vi "Event Handler.vi"(0 "uService Template in":refnum<class "TCP Writer.lvclass">, 5 "Event type":T1=enum."Message", 7 "Item Name":string, 9 "Data":variant, 11 "error in (no error)":errorcluster) -> (4 "uService Template out":refnum<class "TCP Writer.lvclass">, 15 "error out":errorcluster)   [LabVIEW 2026, in "TALOS.lvlib" / "TCP Writer.lvlib" / "TCP Writer.lvclass"]
uses:
  TCP Writer.lvclass
  C:/LabVIEW Code/TALOS/talos/Father of all uServices/Father of all uServices/Father of all uServices.lvclass
  Father of all uServices/Father of all uServices/Event Handler Items.ctl
  Ancestor/Ancestor/Ancestor.lvclass/Ancestor.ctl
  TCP Writer Consumer Case Selector.ctl
  Father of all uServices/Father of all uServices Messages/Consumer Msg/Consumer Msg.lvclass/Consumer Msg.ctl
  FGV/Error Memory/Get Error Description.vi
  Support VIs/Get PC name.vi
  Ancestor/Ancestor/Read ID.vi
  Support VIs/Get Class Name.vi
  <vilib>/Utility/error.llb/Clear Errors.vi
  Father of all uServices/Father of all uServices Messages/Consumer Msg/Send Consumer.vi
  Support VIs/Substitute Error.vi
  FGV/Error Memory/Error Memory Core.vi
  <vilib>/AdvancedString/Delimited String to 1D String Array.vi
  <vilib>/AdvancedString/Delimited String to 1D String Array (string).vi
  Support VIs/Circus Root Path.vi
  FGV/Error Memory/Error Crt Lvl checker.vi
  FGV/Error Memory/Error Memory Core.vi/40c8088d-b597-4017-91af-faa98e00292e.vi
  FGV/Error Memory/Error Memory Core.vi/d4a3ab98-063c-4e44-b43d-fbdcfe6c2be2.vi
  Father of all uServices/Father of all uServices/Father of all uServices.lvclass
  C:/LabVIEW Code/TALOS/builds/Actor Framework PPL/Actor Framework.lvlibp/1abvi3w/vi.lib/ActorFramework/Actor/Actor.lvclass
  Support VIs/Global Memory.vi
  <vilib>/Utility/LVClass/Get LV Class Name.vi
  Support VIs/Is in Packed Library.vi
  Support VIs/TALOS Root path.vi
  Support VIs/Read CSV worksheet.vi
  Support VIs/Global Constants.vi
  <vilib>/Utility/error.llb/General Error Handler.vi
  builds/Actor Framework PPL/Actor Framework.lvlibp/1abvi3w/vi.lib/ActorFramework/Actor/Read Self Enqueuer.vi
  <userlib>/_OpenG.lib/lvdata/lvdata.llb/Get Strings from Enum__ogtk.vi
  builds/Actor Framework PPL/Actor Framework.lvlibp/1abvi3w/vi.lib/ActorFramework/Message Enqueuer/Enqueue.vi
  Support VIs/Error Log.vi
  Ancestor/Ancestor/Ancestor.lvclass
  <vilib>/Comparison/Equal/Equal Functor/Equal Functor.lvclass
  Father of all uServices/Father of all uServices Messages/Consumer Msg/Consumer Msg.lvclass
  TALOS.lvlib
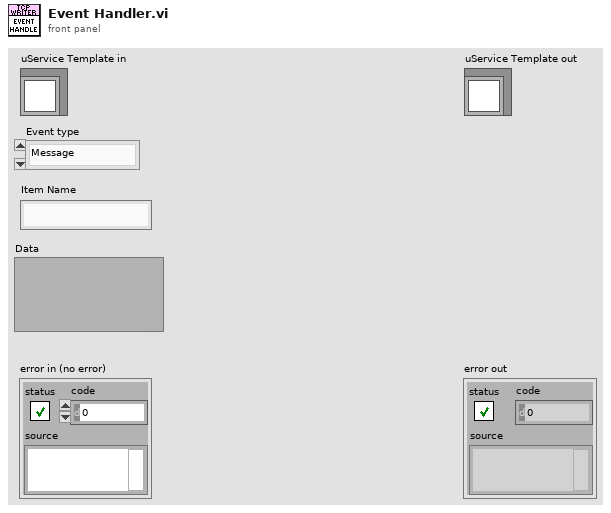
[diagram p1: front panel]
types:
  T1 = typedef "TALOS.lvlib/Father of all uServices.lvlib/Father of all uServices.lvclass/Event Handler Items.ctl" = enum16{"Button Pressed", "Message", "Ready to launch?", "Safe Mode", "Start RUN", "Stop RUN"}
  T2 = typedef "TALOS.lvlib/TCP Writer.lvlib/TCP Writer.lvclass/TCP Writer Consumer Case Selector.ctl" = enum16{"Send message", "Idle", "Check Connection", "Open connection", "Set Client ID"}
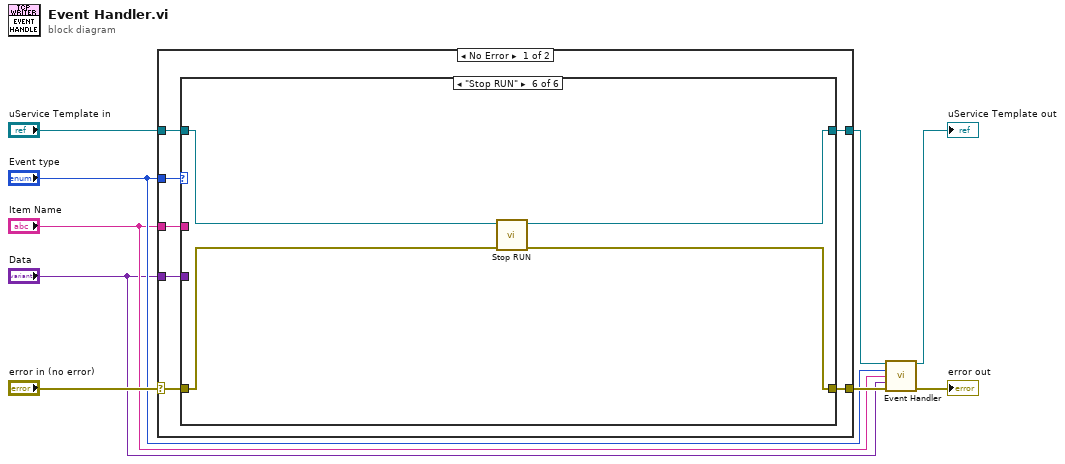
[diagram p0: block diagram]
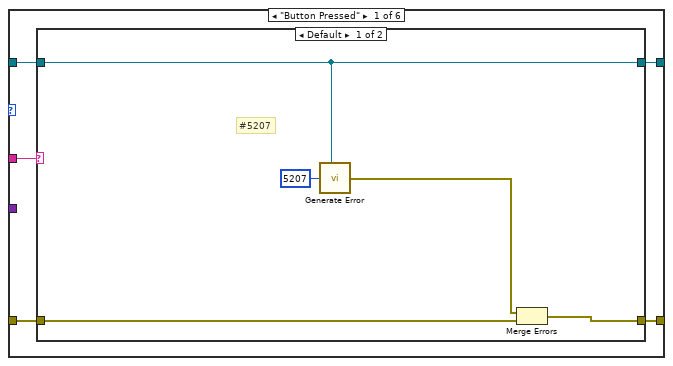
[diagram p2: hidden frame]
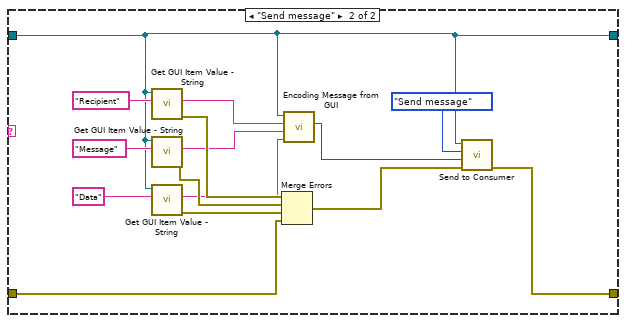
[diagram p3: hidden frame]
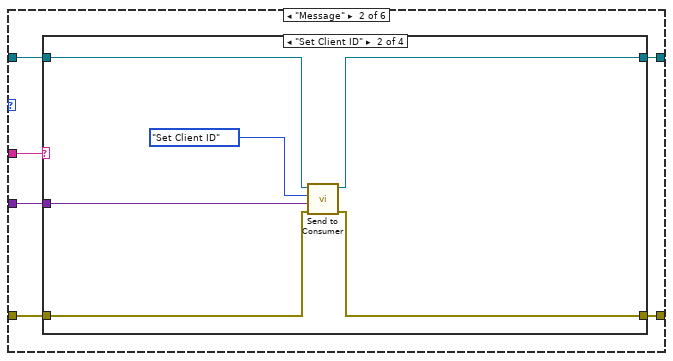
[diagram p4: hidden frame]
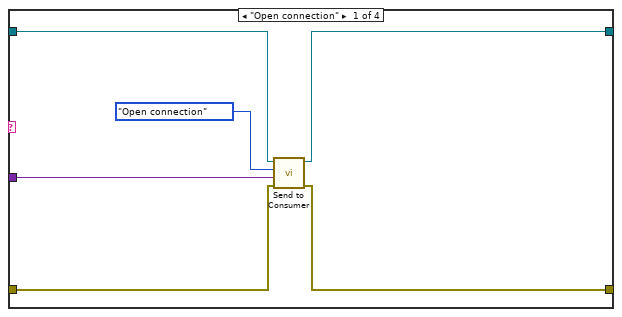
[diagram p5: hidden frame]
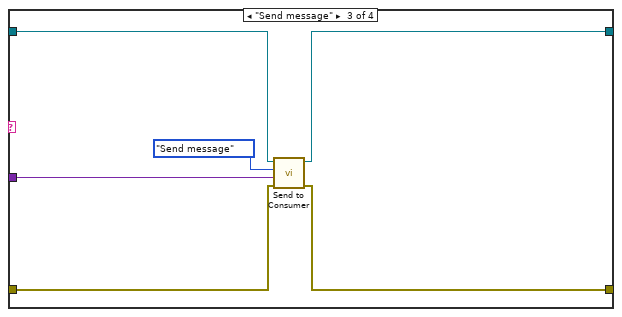
[diagram p6: hidden frame]
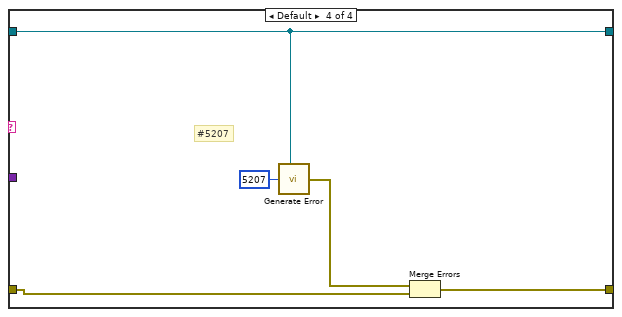
[diagram p7: hidden frame]
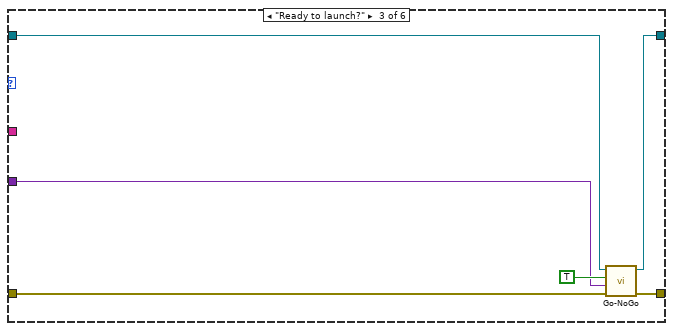
[diagram p8: hidden frame]
diagram:
  n1 = case shown="No Error" "error in (no error)" {
    selector: "error in (no error)" -> [w13 w86]
    tunnel: [w12 w86] -> w7
    tunnel: "uService Template in" -> [w15 w85]
    tunnel: [w14 w85] -> w4
    tunnel: "Event type" -> [w16 _]
    tunnel: "Item Name" -> [w11 _]
    tunnel: "Data" -> [w10 _]
    frame No Error {
      n2 = case shown="\"Stop RUN\"" w16 {
        tunnel: w15 -> [w21 w47 w73 w78 w80 w84]
        tunnel: [w20 w43 w76 w78 w80 w82] -> w14
        tunnel: w13 -> [w17 w44 w74 w77 w79 w83]
        tunnel: [w18 w42 w75 w77 w79 w81] -> w12
        tunnel: w11 -> [w19 w46 _ _ _ _]
        tunnel: w10 -> [_ w45 w71 _ _ _]
        frame "Button Pressed" {
          n3 = case shown="Default" w19 {
            tunnel: w21 -> [w22 w31]
            tunnel: [w22 w31] -> w20
            tunnel: [w25 w32] -> w18
            tunnel: w17 -> [w26 w34]
            frame Default {
              # "#5207"
              n4 = call "Generate Error.vi"("Class"=w22, "Error Code"=5207) -> ("error out"=w24:errorcluster)  [unwired: 5 in]
              n5 = Merge Errors(w24, w26) -> (w25:errorcluster)
            }
            frame "Send message" {
              n6 = call "Get GUI Item Value - String.vi"("FP Item Name"="Recipient", "uService Template in"=w31) -> ("error out"=w37:errorcluster, "Value"=w30:string)  [unwired: 7 in, 1 out]
              n7 = call "Get GUI Item Value - String.vi"("FP Item Name"="Message", "uService Template in"=w31) -> ("error out"=w36:errorcluster, "Value"=w29:string)  [unwired: 7 in, 1 out]
              n8 = call "Get GUI Item Value - String.vi"("FP Item Name"="Data", "uService Template in"=w31) -> ("error out"=w35:errorcluster, "Value"=w28:string)  [unwired: 7 in, 1 out]
              n9 = Merge Errors(w37, w36, w35, w34) -> (w33:errorcluster)
              n10 = call-dynamic "Encoding Message from GUI.vi"("Data"=w28, "Message"=w29, "uS/GD ID"=w30, "uService Template in"=w31) -> ("Variant"=w27:variant)  [unwired: 6 in, 1 out]
              n11 = call "Send to Consumer.vi"("error in (no error)"=w33, "Data"=w27, "Case ID"=TCP_Writer_Consumer_Case_Selector."Send message" ("TCP Listener Consumer Case Selector"), "uService Template in"=w31) -> ("error out"=w32:errorcluster)  [unwired: 6 in, 1 out]
            }
          }
        }
        frame "Message" {
          n12 = case shown="\"Set Client ID\"" w46 {
            tunnel: w47 -> [w53 w59 w65 w68]
            tunnel: w45 -> [w49 w55 w61 _]
            tunnel: w44 -> [w51 w57 w63 w66]
            tunnel: [w52 w58 w64 w68] -> w43
            tunnel: [w50 w56 w62 w67] -> w42
            frame "Open connection" {
              n13 = call "Send to Consumer.vi"("error in (no error)"=w51, "Data"=w49, "Case ID"=TCP_Writer_Consumer_Case_Selector."Open connection" ("TCP Listener Consumer Case Selector"), "uService Template in"=w53) -> ("error out"=w50:errorcluster, "uService Template out"=w52:refnum<class "TCP Writer.lvclass">)  [unwired: 6 in]
            }
            frame "Set Client ID" {
              n14 = call "Send to Consumer.vi"("error in (no error)"=w57, "Data"=w55, "Case ID"=TCP_Writer_Consumer_Case_Selector."Set Client ID" ("TCP Listener Consumer Case Selector"), "uService Template in"=w59) -> ("error out"=w56:errorcluster, "uService Template out"=w58:refnum<class "TCP Writer.lvclass">)  [unwired: 6 in]
            }
            frame "Send message" {
              n15 = call "Send to Consumer.vi"("error in (no error)"=w63, "Data"=w61, "Case ID"=TCP_Writer_Consumer_Case_Selector."Send message" ("TCP Listener Consumer Case Selector"), "uService Template in"=w65) -> ("error out"=w62:errorcluster, "uService Template out"=w64:refnum<class "TCP Writer.lvclass">)  [unwired: 6 in]
            }
            frame Default {
              # "#5207"
              n16 = call "Generate Error.vi"("Class"=w68, "Error Code"=5207) -> ("error out"=w69:errorcluster)  [unwired: 5 in]
              n17 = Merge Errors(w69, w66) -> (w67:errorcluster)
            }
          }
        }
        frame "Ready to launch?" {
          n18 = call-dynamic "Go-NoGo.vi"("error in (no error)"=w74, "Go-NoGo Data"=w71, "Go?"=TRUE, "Father of all uServices in"=w73) -> ("error out"=w75:errorcluster, "Father of all uServices out"=w76:refnum<class "TCP Writer.lvclass">)  [unwired: 6 in]
        }
        frame "Safe Mode" {
        }
        frame "Start RUN" {
        }
        frame "Stop RUN" {
          n19 = call-dynamic "Stop RUN.vi"("error in (no error)"=w83, "TCP Writer in"=w84) -> ("error out"=w81:errorcluster, "TCP Writer out"=w82:refnum<class "TCP Writer.lvclass">)  [unwired: 8 in]
        }
      }
    }
    frame Error {
    }
  }
  n20 = call-parent "Event Handler.vi"("uService Template in"=w4, "Event type"="Event type", "Item Name"="Item Name", "Data"="Data", "error in (no error)"=w7) -> ("uService Template out"=→"uService Template out":refnum<class "TCP Writer.lvclass">, "error out"=→"error out":errorcluster)  [unwired: 9 in]
